vi "Assignment_1_Comparator.vi"() -> ()   [LabVIEW 2019]
panel:
  out "Result":bool
  out "Result":bool
  out "Result":bool
  out "Result":bool
  out "Result":bool
  out "Result":string
  in  "LED":bool
  out "min(x,y)":dbl
  out "max(x,y)":dbl
  in  "y":dbl
  in  "x":dbl
  in  "Num 9":dbl
  in  "Num 8":dbl
  in  "Num 7":dbl
  in  "Num 6":dbl
  in  "Num 5":dbl
  in  "Num 3":dbl
  in  "Num 4":dbl
  out "Result":bool
  in  "Num 2":dbl
  in  "Num 1":dbl
  # "Diagram Disabled Structure is used"
  # "Greater and Less Comparator"
  # "Equal and Not Equal Comparator"
  # "Greater or Equal and Less or Equal Comparator"
  # "Equal to 0 and Not Equal to 0 Comparator"
  # "Greater or Equal to 0 and Less or Equal to 0 Comparator"
  # "Greater than 0 and Less than 0 Comparator"
  # "Max and Min Comparator"
  # "Select Comparator"
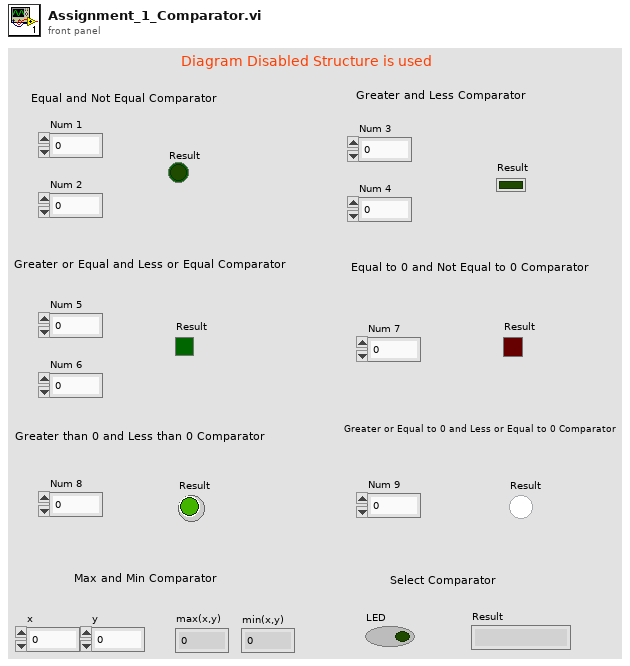
[diagram p1: front panel]
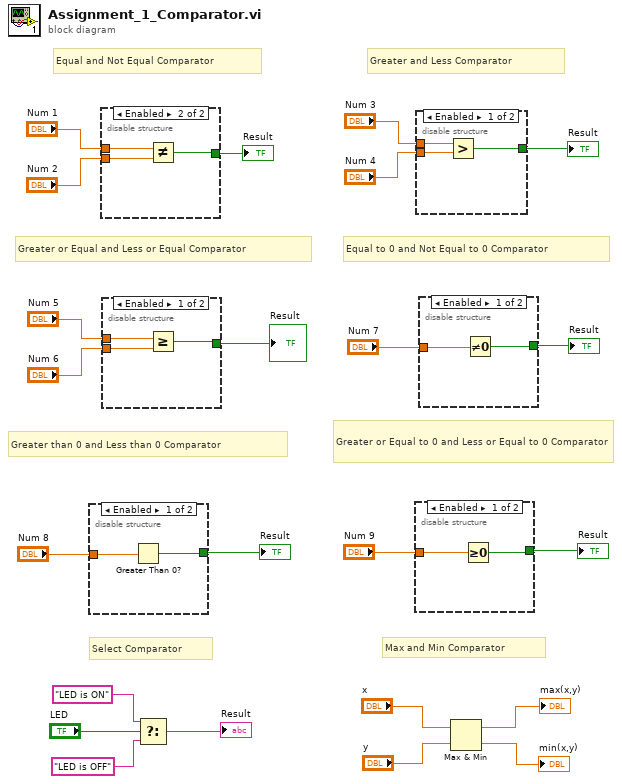
[diagram p0: block diagram]
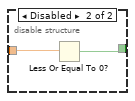
[diagram p2: hidden frame]
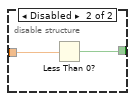
[diagram p3: hidden frame]
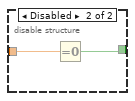
[diagram p4: hidden frame]
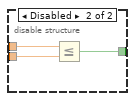
[diagram p5: hidden frame]
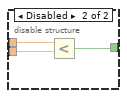
[diagram p6: hidden frame]
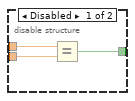
[diagram p7: hidden frame]
diagram:
  # "Select Comparator"
  # "Max and Min Comparator"
  # "Greater or Equal to 0 and Less or Equal to 0 Comparator"
  # "Greater than 0 and Less than 0 Comparator"
  # "Equal to 0 and Not Equal to 0 Comparator"
  # "Greater or Equal and Less or Equal Comparator"
  # "Greater and Less Comparator"
  # "Equal and Not Equal Comparator"
  n1 = disable-structure shown="Enabled" {
    disable-tunnel: "Num 8" -> [w25 w27]
    disable-tunnel: [w24 w26] -> w3
    frame Enabled {
      n2 = Greater Than 0?(x=w25) -> (x > 0?=w24:bool)
    }
    frame Disabled {
      n3 = Less Than 0?(x=w27) -> (x < 0?=w26:bool)
    }
  }
  "Result" <- w3
  n4 = disable-structure shown="Enabled" {
    disable-tunnel: "Num 1" -> [w30 w33]
    disable-tunnel: "Num 2" -> [w29 w32]
    disable-tunnel: [w28 w31] -> w21
    frame Disabled {
      n5 = Equal?(x=w30, y=w29) -> (x = y?=w28:bool)
    }
    frame Enabled {
      n6 = Not Equal?(x=w33, y=w32) -> (x != y?=w31:bool)
    }
  }
  "Result" <- w21
  n7 = disable-structure shown="Enabled" {
    disable-tunnel: "Num 5" -> [w36 w39]
    disable-tunnel: "Num 6" -> [w35 w38]
    disable-tunnel: [w34 w37] -> w1
    frame Enabled {
      n8 = Greater Or Equal?(x=w36, y=w35) -> (x >= y?=w34:bool)
    }
    frame Disabled {
      n9 = Less Or Equal?(x=w39, y=w38) -> (x <= y?=w37:bool)
    }
  }
  "Result" <- w1
  n10 = Select(t="LED is ON", s="LED", f="LED is OFF") -> (s? t:f=→"Result":string)
  n11 = disable-structure shown="Enabled" {
    disable-tunnel: "Num 9" -> [w41 w43]
    disable-tunnel: [w40 w42] -> w2
    frame Enabled {
      n12 = Greater Or Equal To 0?(x=w41) -> (x >= 0?=w40:bool)
    }
    frame Disabled {
      n13 = Less Or Equal To 0?(x=w43) -> (x <= 0?=w42:bool)
    }
  }
  "Result" <- w2
  n14 = disable-structure shown="Enabled" {
    disable-tunnel: "Num 3" -> [w46 w49]
    disable-tunnel: "Num 4" -> [w45 w48]
    disable-tunnel: [w44 w47] -> w5
    frame Enabled {
      n15 = Greater?(x=w46, y=w45) -> (0:w44:bool)
    }
    frame Disabled {
      n16 = Less?(x=w49, y=w48) -> (x < y?=w47:bool)
    }
  }
  "Result" <- w5
  n17 = disable-structure shown="Enabled" {
    disable-tunnel: "Num 7" -> [w51 w53]
    disable-tunnel: [w50 w52] -> w4
    frame Enabled {
      n18 = Not Equal To 0?(x=w51) -> (x != 0?=w50:bool)
    }
    frame Disabled {
      n19 = Equal To 0?(x=w53) -> (x = 0?=w52:bool)
    }
  }
  "Result" <- w4
  n20 = Max & Min(x="x", y="y") -> (max(x,y)=→"max(x,y)":dbl, min(x,y)=→"min(x,y)":dbl)
